vi "Add person.vi"(8 "Error In":errorcluster caption="错误输入", 11 "connection reference":T1) -> (0 "Error Out":errorcluster caption="错误输出", 3 "Patient_ID":i64)   [LabVIEW 2015, in "Sample.lvlib"]
uses:
  Sample.lvlib
  <vilib>/addons/database/Connection.llb/Conn ObjectReference.ctl
  Support/Add Person State.ctl
  Sub VIs/Database Processing/Support/Table/personal_information.ctl
  Sub VIs/Database Processing/Database Processing.lvlib
  <vilib>/addons/database/NI_Database_API.lvlib
panel:
  in  "Cancel":bool
  in  "Add":bool
  in  "出生日期":string
  in  "性别":string
  in  "姓名":string
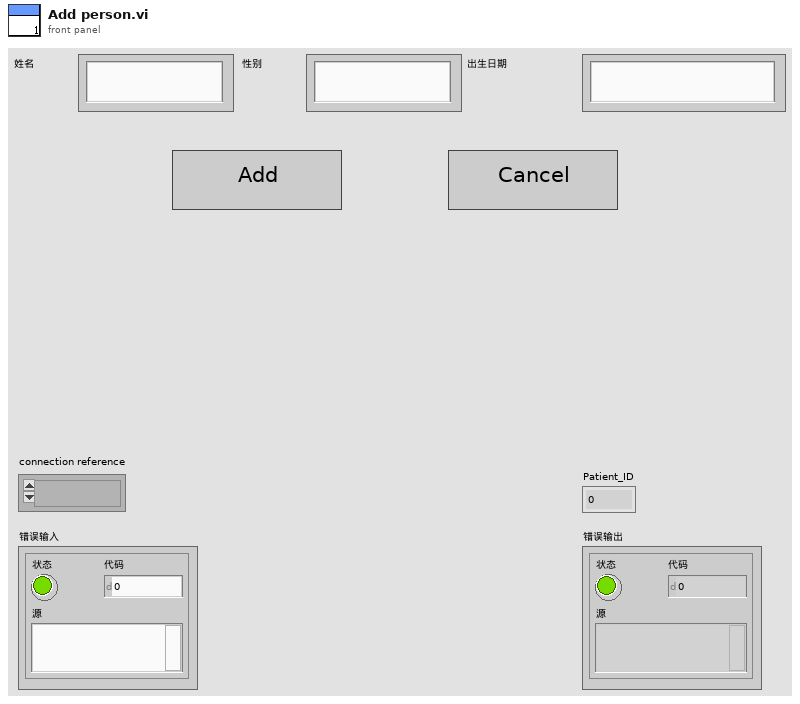
[diagram p1: front panel]
types:
  T1 = typedef "NI_Database_API.lvlib/Conn ObjectReference.ctl" = refnum<k1>
  T2 = typedef "Database Processing.lvlib/personal_information.ctl" = cluster{"Patient_ID":i64, "name":string, "sex":string, "birthday":string}
  T3 = typedef "Sample.lvlib/Add Person State.ctl" = enum16{"Initialize", "Connect Database", "Wait For Event", "Add", "Cancel", "Exit", "Get Patient_ID"}
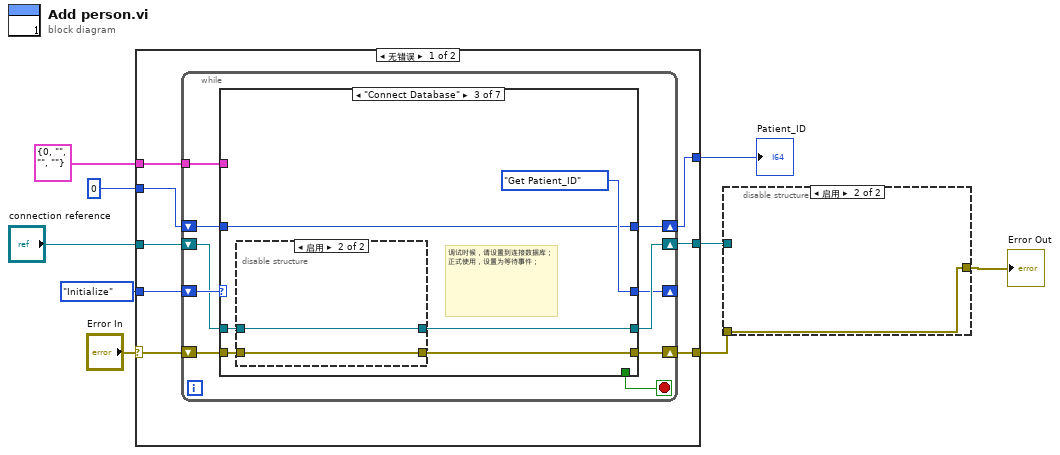
[diagram p0: block diagram]
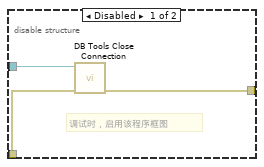
[diagram p2: hidden frame]
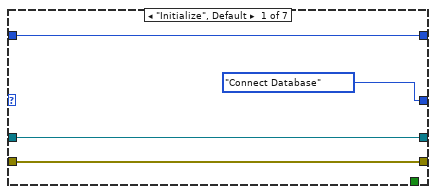
[diagram p3: hidden frame]
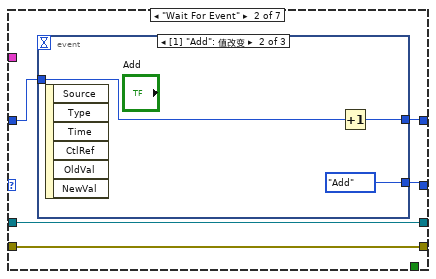
[diagram p4: hidden frame]
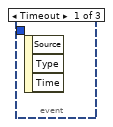
[diagram p5: hidden frame]
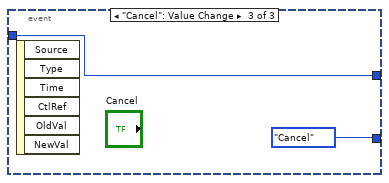
[diagram p6: hidden frame]
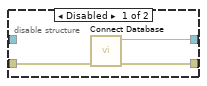
[diagram p7: hidden frame]
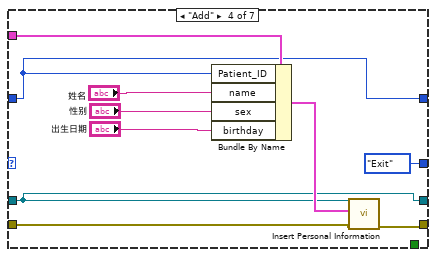
[diagram p8: hidden frame]
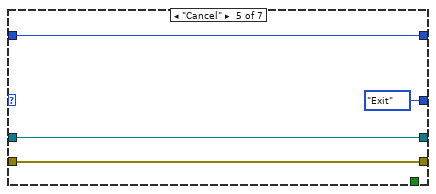
[diagram p9: hidden frame]
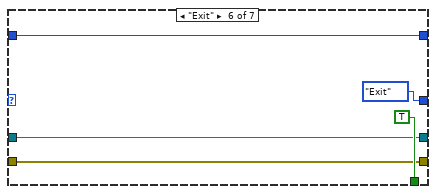
[diagram p10: hidden frame]
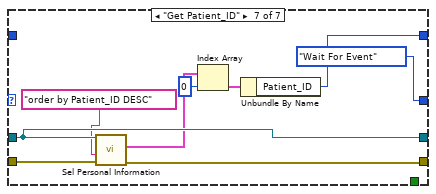
[diagram p11: hidden frame]
diagram:
  n1 = case shown="无错误" "Error In" {
    selector: "Error In" -> [w15 w83]
    tunnel: Add_Person_State."Initialize" ("State") -> [w17 _]
    tunnel: "connection reference" -> [w16 w82]
    tunnel: [w14 w82] -> w6
    tunnel: [w13 w83] -> w5
    tunnel: i64 0 ("Patient_ID") -> [w12 w81]
    tunnel: T2 {"Patient_ID"=0, "name"="", "sex"="", "birthday"=""} ("personal_information") -> [w11 _]
    tunnel: [w10 w81] -> w2
    frame No Error {
      n2 = while {
        shift-right: [w24] -> _
        shift-left: w17 -> [w27]
        shift-right: [w26] -> w14
        shift-left: w16 -> [w25]
        shift-right: [w22] -> w13
        shift-left: w15 -> [w23]
        shift-right: [w20] -> w10
        shift-left: w12 -> [w19]
        tunnel: w11 -> [w18]
        stop <- w21 stop-if-true
        n3 = case shown="\"Connect Database\"" w27 {
          tunnel: [w31 w36 w45 w53 w66 w70 w79] -> w26
          tunnel: w25 -> [w31 w36 w44 w53 w66 w70 w79]
          tunnel: [Add_Person_State."Connect Database" ("State") w35 Add_Person_State."Get Patient_ID" ("State") Add_Person_State."Exit" ("State") Add_Person_State."Exit" ("State") Add_Person_State."Exit" ("State") Add_Person_State."Wait For Event" ("State")] -> w24
          tunnel: w23 -> [w29 w34 w46 w56 w64 w68 w77]
          tunnel: [w29 w34 w43 w55 w64 w68 w76] -> w22
          tunnel: [_ _ _ _ _ TRUE _] -> w21
          tunnel: [w28 w33 w42 w60 w63 w67 w72] -> w20
          tunnel: w19 -> [w28 w32 w42 w60 w63 w67 _]
          tunnel: w18 -> [_ _ _ w61 _ _ _]
          frame "Initialize", Default {
          }
          frame "Wait For Event" {
            n4 = event shown="[1] \"Add\": 值改变" {
              selector: _ -> [_ _ _]
              dyn-events: _ -> [_ _ _]
              timeout: _ -> [_ _ _]
              tunnel: [_ Add_Person_State."Add" ("State") Add_Person_State."Cancel" ("State")] -> w35
              tunnel: [_ w38 w40] -> w33
              tunnel: w32 -> [_ w37 w40]
              event Timeout {
                n5 = event-data() -> ()  [unwired: 1 in, 3 out]
              }
              event "Add": Value Change {
                n6 = event-data() -> ()  [unwired: 1 in, 6 out]
                n7 = Increment(x=w37) -> (x+1=w38:i64)
              }
              event "Cancel": Value Change {
                n8 = event-data() -> ()  [unwired: 1 in, 6 out]
              }
            }
          }
          frame "Connect Database" {
            # "调试时候，请设置到连接数据库；\n正式使用，设置为等待事件；"
            n9 = disable-structure shown="启用" {
              disable-tunnel: w46 -> [w50 w51]
              disable-tunnel: [w49 w51] -> w43
              disable-tunnel: [w48 w52] -> w45
              disable-tunnel: w44 -> [_ w52]
              frame Disabled {
                n10 = call "Connect Database.vi"("error in (no error)"=w50) -> ("error out"=w49:errorcluster, "connection reference"=w48:T1)  [unwired: 9 in]
              }
              frame Enabled {
              }
            }
          }
          frame "Add" {
            n11 = Bundle By Name(cluster=w61, "Patient_ID"=w60, "name"="姓名", "sex"="性别", "birthday"="出生日期") -> (w54:T2)
            n12 = call "Insert Personal Information.vi"("error in (no error)"=w56, "personal_information Input"=w54, "connection reference"=w53) -> ("error out"=w55:errorcluster)  [unwired: 8 in]
          }
          frame "Cancel" {
          }
          frame "Exit" {
          }
          frame "Get Patient_ID" {
            n13 = call "Sel Personal Information.vi"("error in (no error)"=w77, "condition"="order by Patient_ID DESC" ("Condition"), "connection reference"=w79) -> ("error out"=w76:errorcluster, "personal information"=w75:T2[])  [unwired: 7 in]
            n14 = Index Array(array=w75, index=0 ("索引")) -> (element=w73:T2)
            n15 = Unbundle By Name(w73) -> ("Patient_ID"=w72:i64)
          }
        }
      }
    }
    frame Error {
    }
  }
  "Patient_ID" <- w2
  n16 = disable-structure shown="启用" {
    disable-tunnel: w6 -> [w86 _]
    disable-tunnel: w5 -> [w85 w87]
    disable-tunnel: [w84 w87] -> w1
    frame Disabled {
      # "调试时，启用该程序框图"
      n17 = call <vilib>:"DB Tools Close Connection.vi"("error in (no error)"=w85, "connection reference"=w86) -> ("error out"=w84:errorcluster)  [unwired: 5 in]
    }
    frame Enabled {
    }
  }
  "Error Out" <- w1
